vi "Chronometer_.vi"(7 "Time in eclipse (s)":dbl=2122.0 format="%#_13g", 9 "Action":enum16{"Count", "Stop", "Reset"}(ring)) -> (0 "Minute":i32, 1 "Hour":i32, 2 "Action out":enum16{"Count", "Stop", "Reset"}(ring), 3 "Boolean":bool, 4 "Fractional Second":dbl format="%#.4g", 6 "Second":i32)   [LabVIEW 2015]
uses:
  utilities/Test_Code/Global 5.vi
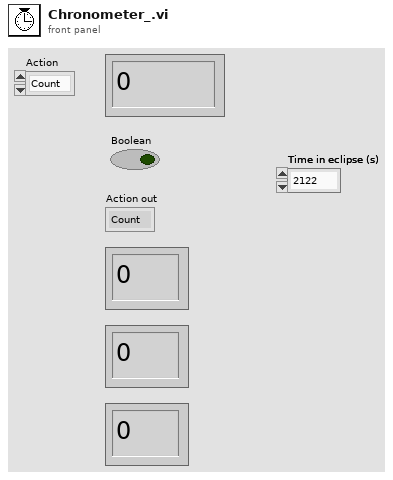
[diagram p1: front panel]
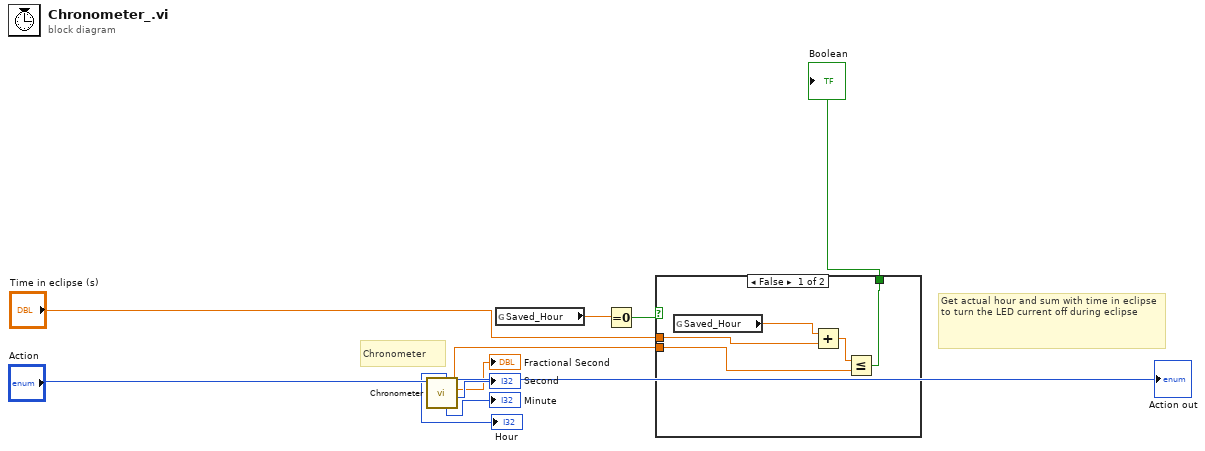
[diagram p0: block diagram]
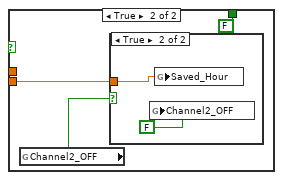
[diagram p2: hidden frame]
diagram:
  # "Get actual hour and sum with time in eclipse to turn the LED current off during eclipse"
  # "Chronometer"
  n1 = call "Chronometer.vi"("Action in"="Action") -> ("Second"=→"Second":i32, "Fractional Second"=→"Fractional Second":dbl, "Time"=w2:dbl, "Minute"=→"Minute":i32, "Hour"=→"Hour":i32, "Action out"=→"Action out":enum16{"Count", "Stop", "Reset"})  [unwired: 5 in]
  n2 = global read "Global 5.vi" "Saved_Hour"() -> (w4:dbl)
  n3 = Equal To 0?(x=w4) -> (x = 0?=w3:bool)
  n4 = case shown="False" w3 {
    tunnel: w2 -> [w14 w18]
    tunnel: [w16 FALSE] -> w11
    tunnel: "Time in eclipse (s)" -> [w12 _]
    frame False {
      n5 = global read "Global 5.vi" "Saved_Hour"() -> (w13:dbl)
      n6 = Add(x=w13, y=w12) -> (x+y=w15:dbl)
      n7 = Less Or Equal?(x=w15, y=w14) -> (x <= y?=w16:bool)
    }
    frame True {
      n8 = global read "Global 5.vi" "Channel2_OFF"() -> (w19:bool)
      n9 = case shown="True" w19 {
        tunnel: w18 -> [_ w20]
        frame False {
        }
        frame True {
          n10 = global write "Global 5.vi" "Channel2_OFF"(FALSE ("Channel2")) -> ()
          n11 = global write "Global 5.vi" "Saved_Hour"(w20) -> ()
        }
      }
    }
  }
  "Boolean" <- w11
